vi "init.vi"(0 "FixedFrameBuilder in":refnum<class "FixedFrameBuilder.lvclass">, 5 "Address":u8, 7 "Function":u8, 9 "DataSize":i32, 11 "error in (no error)":errorcluster) -> (4 "FixedFrameBuilder out":refnum<class "FixedFrameBuilder.lvclass">, 15 "error out":errorcluster)   [LabVIEW 2016, in "FixedFrameBuilder.lvclass"]
uses:
  FixedFrameBuilder.lvclass
  Common_RT_Utilities/U8ArrayBuilderManualIndexing/U8ArrayBuilderManualIndexing.lvclass
  FixedFrameBuilder.lvclass/FixedFrameBuilder.ctl
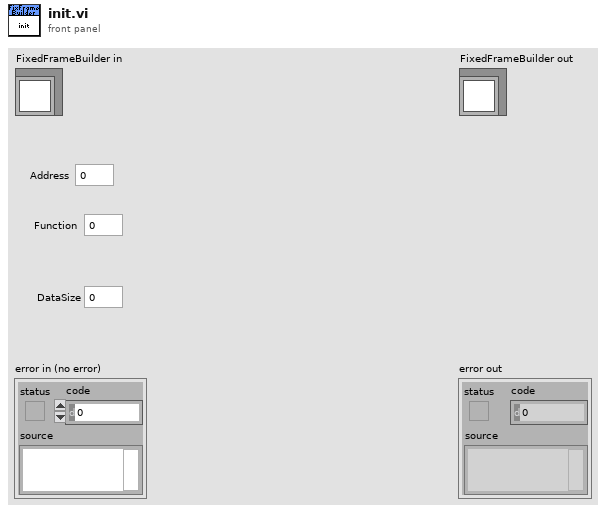
[diagram p1: front panel]
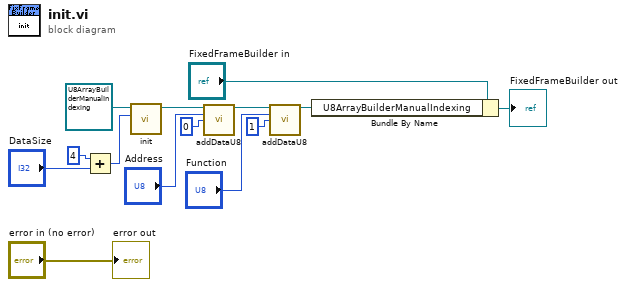
[diagram p0: block diagram]
diagram:
  n1 = Add(x=4, y="DataSize") -> (x+y=w8:i32)
  n2 = call "init.vi"("Size"=w8, "U8ArrayBuilderManualIndexing in"=refnum<class "U8ArrayBuilderManualIndexing.lvclass"> refnum ("RTUtilities.lvlib:U8ArrayBuilderManualIndexing.lvclass")) -> ("U8ArrayBuilderManualIndexing out"=w3:refnum<class "U8ArrayBuilderManualIndexing.lvclass">)  [unwired: 8 in, 1 out]
  n3 = call "addDataU8.vi"("U8ArrayBuilderManualIndexing in"=w3, "Data"="Address", "Index"=0 ("index")) -> ("U8ArrayBuilderManualIndexing out"=w2:refnum<class "U8ArrayBuilderManualIndexing.lvclass">)  [unwired: 10 in, 2 out]
  n4 = call "addDataU8.vi"("U8ArrayBuilderManualIndexing in"=w2, "Data"="Function", "Index"=1 ("index")) -> ("U8ArrayBuilderManualIndexing out"=w1:refnum<class "U8ArrayBuilderManualIndexing.lvclass">)  [unwired: 10 in, 2 out]
  n5 = Bundle By Name(cluster="FixedFrameBuilder in", "U8ArrayBuilderManualIndexing"=w1) -> (→"FixedFrameBuilder out":refnum<class "FixedFrameBuilder.lvclass">)
  "error out" <- "error in (no error)"
